vi "Stop Core.vi"(10 "final error code":i32, 11 "SCADA in":refnum<class "EMS.lvclass">) -> (3 "SCADA out":refnum<class "EMS.lvclass">)   [LabVIEW 2018, in "EMS Core.lvlib" / "EMS.lvclass"]
doc: "(<B>Filename</B>: Actor Framework.lvlib:Actor.lvclass:Stop Core.vi)\n\nDefines what the actor does before it stops. Use the <B>final error code</B> input to determine whether the actor shut down in response to an error.\n\nBy default, this method does nothing. A descendant class may override it to define behavior, such as shutting down any processes the actor initiated in its override of the Actor Core method."
uses:
  EMS.lvclass
  Controls/Microgrid State.ctl
  <vilib>/ActorFramework/Time-Delayed Send Message/Time-Delay Override Options.ctl
  EMS.lvclass/EMS.ctl
  <vilib>/ActorFramework/Message Enqueuer/Message Enqueuer.lvclass/Message Enqueuer.ctl
  <vilib>/ActorFramework/Message Enqueuer/Enqueue.vi
  <vilib>/ActorFramework/Stop Msg/Stop Msg.lvclass
  C:/Program Files (x86)/National Instruments/LabVIEW 2018/vi.lib/ActorFramework/Message/Message.lvclass
  <vilib>/ActorFramework/Message Priority Queue/Priority Enqueue.vi
  EMS Generic Actor/EMS Generic/EMS Generic.lvclass
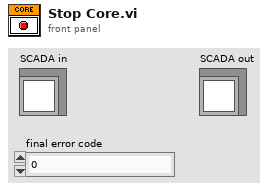
[diagram p1: front panel]
types:
  T1 = typedef "Time-Delay Override Options.ctl" = enum16{"Send next copy now", "Skip next scheduled copy", "Send next copy now and stop all further copies", "Stop all further copies"}
  T2 = typedef "EMS Core.lvlib/EMS.lvclass/Microgrid State.ctl" = enum16{"Discovery", "Commissioning", "Activation", "Blackstart", "OnGrid", "OffGrid", "Island", "Resynchronization", "Manual", "Shutdown", "Stop"}
  T3 = typedef "EMS Core.lvlib/EMS.lvclass/Delivery Notifiers.ctl" = cluster{"Watchdog":refnum<notifier>, "Find and Rejoin":refnum<notifier>}
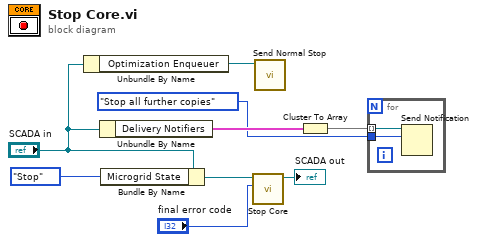
[diagram p0: block diagram]
diagram:
  n1 = Unbundle By Name("SCADA in") -> ("Optimization Enqueuer"=w2:refnum<class "Message Enqueuer.lvclass">)
  n2 = Unbundle By Name("SCADA in") -> ("Delivery Notifiers"=w5:T3)
  n3 = Bundle By Name(cluster="SCADA in", "Microgrid State"=Microgrid_State."Stop") -> (w7:refnum<class "EMS.lvclass">)
  n4 = call-parent "Stop Core.vi"("final error code"="final error code", "EMS Generic in"=w7) -> ("EMS Generic out"=→"SCADA out":refnum<class "EMS.lvclass">)  [unwired: 9 in]
  n5 = call <vilib>:"Send Normal Stop.vi"("Message Enqueuer"=w2) -> ()  [unwired: 10 in, 1 out]
  n6 = Cluster To Array(cluster=w5) -> (array=w1:refnum<notifier>[])
  n7 = for {
    tunnel: Time-Delay_Override_Options."Stop all further copies" ("notification") -> [w11]
    tunnel: w1 -> [w10] mode=indexing
    n8 = Send Notification(notification=w11, notifier=w10) -> ()  [unwired: 1 in, 2 out]
  }
